vi "Spectrum_Test.vi"() -> ()   [LabVIEW 2015]
uses:
  <vilib>/Analysis/2dsp.llb/Real FFT.vi
  <vilib>/Analysis/3filter.llb/Butterworth Filter (DBL).vi
  <vilib>/Analysis/NI_AALBase.lvlib
  <vilib>/Analysis/NI_AALPro.lvlib
panel:
  in  "advanced filter parameters":T1={"passband ripple (dB)"=0.01, "stopband start (Hz)"=0.0, "stopband gain (dB)"=-96.0, "compute filter stopband ? (T)"=TRUE}
  in  "stop":bool
  out "Power Spectrum":cluster{"Elevation":sgl, dbl, dbl[]}(graph)
  in  "BW(MHz)":i32
  in  "Active Antenna":string(combo)="RX1"
  in  "Gain [dB]":dbl=20.0 format="%#.6p"
  in  "Carrier\nFrequency [MHz]":dbl=90500000.0 format="%#.6p"
  in  "IQ Sampling\nRate [S/sec]":dbl=200000.0 format="%#.6p"
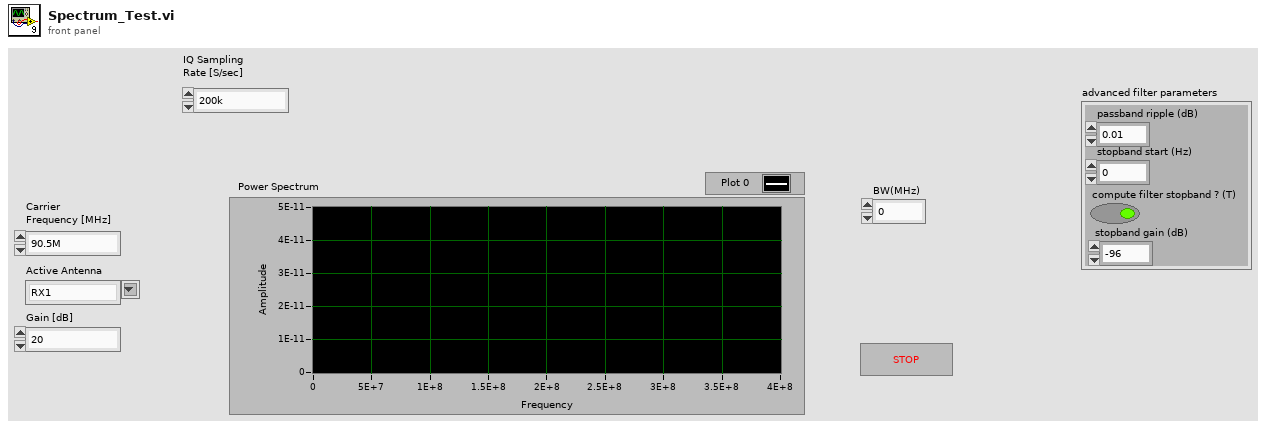
[diagram p1: front panel]
types:
  T1 = cluster{"passband ripple (dB)":dbl, "stopband start (Hz)":dbl, "stopband gain (dB)":dbl, "compute filter stopband ? (T)":bool}
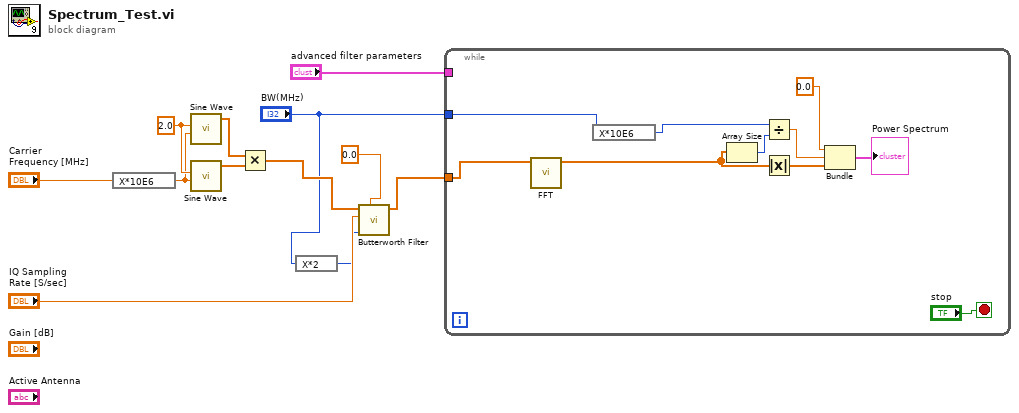
[diagram p0: block diagram]
diagram:
  w9 = 2.0 ("x")
  n1 = expression code="X*10E6"("Carrier\nFrequency [MHz]") -> (w7:dbl)
  n2 = call <vilib>:"Sine Wave.vi"("amplitude"=w9, "frequency"=w7) -> ("sine wave"=w10:dbl[])  [unwired: 3 in, 2 out]
  n3 = call <vilib>:"Sine Wave.vi"("amplitude"=w9, "frequency"=w7) -> ("sine wave"=w11:dbl[])  [unwired: 3 in, 2 out]
  n4 = Multiply(x=w10, y=w11) -> (x*y=w6:dbl[])
  n5 = expression code="X*2"("BW(MHz)") -> (w1:i32)
  n6 = call-poly <vilib>:"Butterworth Filter.vi"("filter type"=sgl 0.0 ("Elevation"), "low cutoff freq: fl"=w1, "sampling freq: fs"="IQ Sampling\nRate [S/sec]", "X"=w6) -> ("Filtered X"=w5:dbl[])  [unwired: 4 in, 1 out]
  n7 = while {
    tunnel: "advanced filter parameters" -> [_]
    tunnel: w5 -> [w15]
    tunnel: "BW(MHz)" -> [w13]
    stop <- "stop" stop-if-true
    n8 = call-poly <vilib>:"FFT.vi"("X"=w15) -> ("FFT {X}"=w17:cdb[])  [unwired: 9 in, 1 out]
    n9 = expression code="X*10E6"(w13) -> (w14:i32)
    n10 = Array Size(array=w17) -> (size(s)=w18:i32)
    n11 = Divide(x=w14, y=w18) -> (x/y=w20:dbl)
    n12 = Absolute Value(x=w17) -> (abs(x)=w19:dbl[])
    n13 = Bundle("Elevation"=sgl 0.0, w20, w19) -> (→"Power Spectrum":cluster{"Elevation":sgl, dbl, dbl[]})  [unwired: 1 in]
  }
